vi "Get Type.vi"(8 "error in (no error)":errorcluster, 11 "Plastic Parts in":refnum<class "Plastic Parts.lvclass">) -> (0 "error out":errorcluster, 2 "Item Type":T1, 3 "Plastic Parts out":refnum<class "Plastic Parts.lvclass">)   [LabVIEW 2020, in "Plastic Parts.lvclass"]
uses:
  Plastic Parts.lvclass
  Item/Item Type.ctl
  Item/Item.lvclass
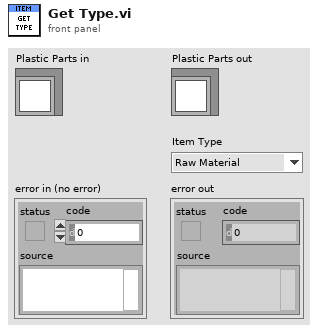
[diagram p1: front panel]
types:
  T1 = typedef "Item.lvclass/Item Type.ctl" = enum16{"Raw Material", "Component", "Module", "Product"}
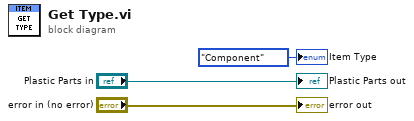
[diagram p0: block diagram]
diagram:
  "error out" <- "error in (no error)"
  "Plastic Parts out" <- "Plastic Parts in"
  "Item Type" <- Item_Type."Component" ("Item Type")
